vi "check out tracking state.vi"(6 "tick count":u32, 8 "ff vel?":bool, 9 "check out state":bool=TRUE, 10 "state number":u8, 11 "previous state":T1={"x state"={"pos estimate"=0.0, "v estimate"=0.0, "weighted position error sum"=0.0, "photon count"=0, "transmit tick count"=0, "axis number"=0, "px (levels^2)"=0.0, "pxv (levels^2/ticks)"=0.0, "pv (levels^2/ticks^2)"=0.0, "vel diff (levels^2/ticks^3)"=0.0, "gx"=0.0, "rtwiddle"=0.0, "photon count ch0"=0, "photon count ch1"=0, "Dx -levels^2/ticks"=0.0}, "y state"={"pos estimate"=0.0, "v estimate"=0.0, "weighted position error sum"=0.0, "photon count"=0, "transmit tick count"=0, "axis number"=1, "px (levels^2)"=0.0, "pxv (levels^2/ticks)"=0.0, "pv (levels^2/ticks^2)"=0.0, "vel diff (levels^2/ticks^3)"=0.0, "gx"=0.0, "rtwiddle"=0.0, "photon count ch0"=0, "photon count ch1"=0, "Dx -levels^2/ticks"=0.0}, "z state"={"pos estimate"=0.0, "v estimate"=0.0, "weighted position error sum"=0.0, "photon count"=0, "transmit tick count"=0, "axis number"=2, "px (levels^2)"=0.0, "pxv (levels^2/ticks)"=0.0, "pv (levels^2/ticks^2)"=0.0, "vel diff (levels^2/ticks^3)"=0.0, "gx"=0.0, "rtwiddle"=0.0, "photon count ch0"=0, "photon count ch1"=0, "Dx -levels^2/ticks"=0.0}, "spot number"=0}) -> (3 "state out":T1={"x state"={"pos estimate"=0.0, "v estimate"=0.0, "weighted position error sum"=0.0, "photon count"=0, "transmit tick count"=0, "axis number"=0, "px (levels^2)"=0.0, "pxv (levels^2/ticks)"=0.0, "pv (levels^2/ticks^2)"=0.0, "vel diff (levels^2/ticks^3)"=0.0, "gx"=0.0, "rtwiddle"=0.0, "photon count ch0"=0, "photon count ch1"=0, "Dx -levels^2/ticks"=0.0}, "y state"={"pos estimate"=0.0, "v estimate"=0.0, "weighted position error sum"=0.0, "photon count"=0, "transmit tick count"=0, "axis number"=1, "px (levels^2)"=0.0, "pxv (levels^2/ticks)"=0.0, "pv (levels^2/ticks^2)"=0.0, "vel diff (levels^2/ticks^3)"=0.0, "gx"=0.0, "rtwiddle"=0.0, "photon count ch0"=0, "photon count ch1"=0, "Dx -levels^2/ticks"=0.0}, "z state"={"pos estimate"=0.0, "v estimate"=0.0, "weighted position error sum"=0.0, "photon count"=0, "transmit tick count"=0, "axis number"=2, "px (levels^2)"=0.0, "pxv (levels^2/ticks)"=0.0, "pv (levels^2/ticks^2)"=0.0, "vel diff (levels^2/ticks^3)"=0.0, "gx"=0.0, "rtwiddle"=0.0, "photon count ch0"=0, "photon count ch1"=0, "Dx -levels^2/ticks"=0.0}, "spot number"=0})   [LabVIEW 2010]
uses:
  kalman 3-axis state.ctl
  integrating single axis kalman state.ctl
  <vilib>/rvi/DataTransferAndStorage/Container/XNode/niFpgaContainer.xnode
  <vilib>/rvi/Memory/Memory_Emulation/nirvimemoryEmulationManagerCache_GetValue.vi
  <vilib>/rvi/DataTransferAndStorage/Container/Common/niFpgaContainerGetUniqueNameForEmu.vi
  <vilib>/rvi/Memory/Memory_Emulation/nirvimemoryEmulationManagerCache_InsertValue.vi
  <vilib>/Utility/error.llb/Clear Errors.vi
  <vilib>/rvi/Memory/Memory_Emulation/nirvimemoryEmulationManagerCache_SetValue.vi
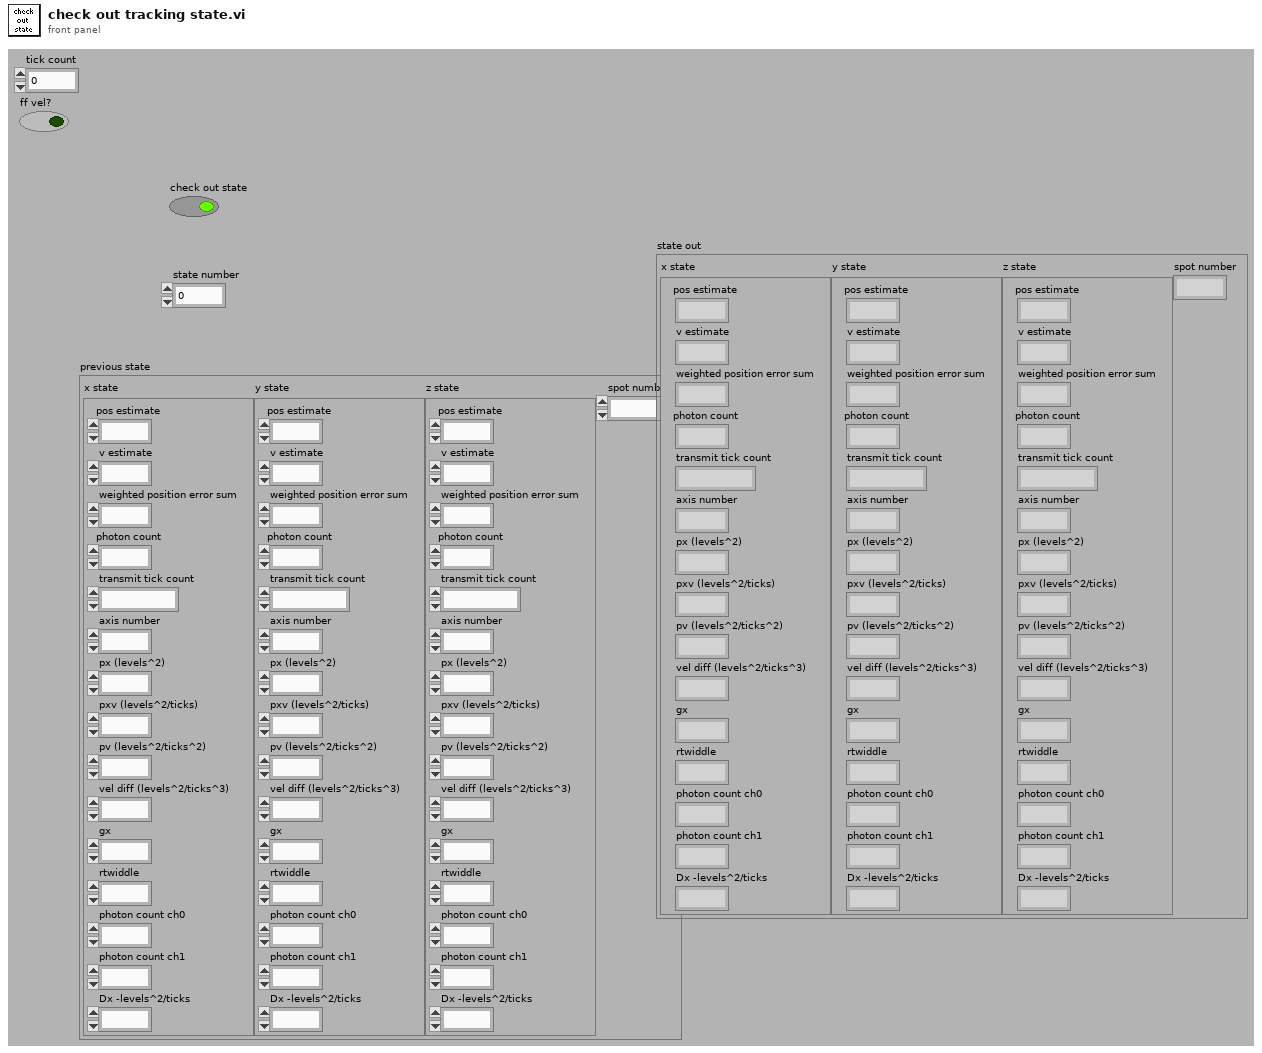
[diagram p1: front panel]
types:
  T1 = typedef "kalman 3-axis state.ctl" = cluster{"x state":T2, "y state":T2, "z state":T2, "spot number":u8}
  T2 = typedef "integrating single axis kalman state.ctl" = cluster{"pos estimate":fxp<+/-,32,16>, "v estimate":fxp<+/-,16,0>, "weighted position error sum":fxp<+/-,32,32>, "photon count":u32, "transmit tick count":u32, "axis number":u8, "px (levels^2)":fxp<+,32,19>, "pxv (levels^2/ticks)":fxp<+,32,2>, "pv (levels^2/ticks^2)":fxp<+,32,-14>, "vel diff (levels^2/ticks^3)":fxp<+,24,-22>, "gx":fxp<+,16,8>, "rtwiddle":fxp<+,16,26>, "photon count ch0":u32, "photon count ch1":u32, "Dx -levels^2/ticks":fxp<+,32,19>}
  T3 = cluster{"x state":cluster{"pos estimate":fxp<+/-,32,16>, "v estimate":fxp<+/-,16,0>, "weighted position error sum":fxp<+/-,32,32>, "photon count":u32, "transmit tick count":u32, "axis number":u8, "px (levels^2)":fxp<+,32,19>, "pxv (levels^2/ticks)":fxp<+,32,2>, "pv (levels^2/ticks^2)":fxp<+,32,-14>, "vel diff (levels^2/ticks^3)":fxp<+,24,-22>, "gx":fxp<+,16,8>, "rtwiddle":fxp<+,16,26>, "photon count ch0":u32, "photon count ch1":u32, "Dx - for pos only k-f":fxp<+,32,19>}, "y state":cluster{"pos estimate":fxp<+/-,32,16>, "v estimate":fxp<+/-,16,0>, "weighted position error sum":fxp<+/-,32,32>, "photon count":u32, "transmit tick count":u32, "axis number":u8, "px (levels^2)":fxp<+,32,19>, "pxv (levels^2/ticks)":fxp<+,32,2>, "pv (levels^2/ticks^2)":fxp<+,32,-14>, "vel diff (levels^2/ticks^3)":fxp<+,24,-22>, "gx":fxp<+,16,8>, "rtwiddle":fxp<+,16,26>, "photon count ch0":u32, "photon count ch1":u32, "Dx - for pos only k-f":fxp<+,32,19>}, "z state":cluster{"pos estimate":fxp<+/-,32,16>, "v estimate":fxp<+/-,16,0>, "weighted position error sum":fxp<+/-,32,32>, "photon count":u32, "transmit tick count":u32, "axis number":u8, "px (levels^2)":fxp<+,32,19>, "pxv (levels^2/ticks)":fxp<+,32,2>, "pv (levels^2/ticks^2)":fxp<+,32,-14>, "vel diff (levels^2/ticks^3)":fxp<+,24,-22>, "gx":fxp<+,16,8>, "rtwiddle":fxp<+,16,26>, "photon count ch0":u32, "photon count ch1":u32, "Dx - for pos only k-f":fxp<+,32,19>}, "spot number":u8}
  T4 = cluster{"pos estimate":fxp<+/-,32,16>, "v estimate":fxp<+/-,16,0>, "weighted position error sum":fxp<+/-,32,32>, "photon count":u32, "transmit tick count":u32, "axis number":u8, "px (levels^2)":fxp<+,32,19>, "pxv (levels^2/ticks)":fxp<+,32,2>, "pv (levels^2/ticks^2)":fxp<+,32,-14>, "vel diff (levels^2/ticks^3)":fxp<+,24,-22>, "gx":fxp<+,16,8>, "rtwiddle":fxp<+,16,26>, "photon count ch0":u32, "photon count ch1":u32, "Dx - for pos only k-f":fxp<+,32,19>}
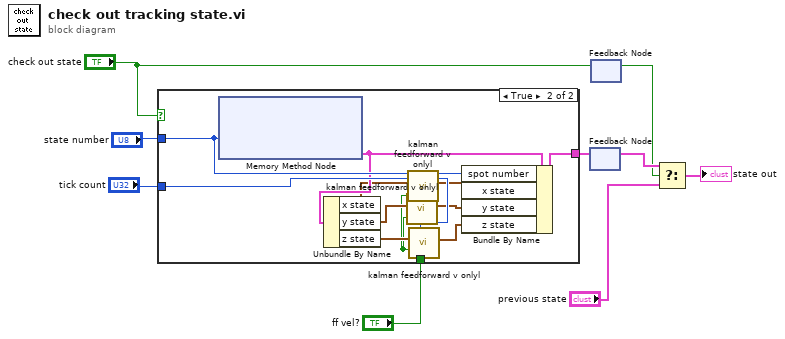
[diagram p0: block diagram]
diagram:
  n1 = case shown="True" "check out state" {
    tunnel: "state number" -> [_ w20]
    tunnel: "tick count" -> [_ w19]
    tunnel: [_ w18] -> w7
    tunnel: "ff vel?" -> [_ w10]
    frame False {
    }
    frame True {
      n2 = xnode ("Memory Method Node")("Address"=w20) -> ("Data"=w17:T3)  [unwired: 1 in, 1 out]
      n3 = Unbundle By Name(w17) -> ("x state"=w16:T4, "y state"=w15:T4, "z state"=w14:T4)
      n4 = call "kalman feedforward v onlyl.vi"("ff vel?"=w10, "tick count"=w19, "state in"=w15) -> ("state out"=w12:T2)  [unwired: 8 in]
      n5 = call "kalman feedforward v onlyl.vi"("ff vel?"=w10, "tick count"=w19, "state in"=w16) -> ("state out"=w13:T2)  [unwired: 8 in]
      n6 = call "kalman feedforward v onlyl.vi"("ff vel?"=w10, "tick count"=w19, "state in"=w14) -> ("state out"=w11:T2)  [unwired: 8 in]
      n7 = Bundle By Name(cluster=w17, "spot number"=w20, "x state"=w13, "y state"=w12, "z state"=w11) -> (w18:T3)
    }
  }
  n8 = feedback-in #1(w7) -> ()
  n9 = feedback #1() -> (w6:T3)  [unwired: 1 in]
  n10 = feedback #2() -> (w2:bool)  [unwired: 1 in]
  n11 = feedback-in #2("check out state") -> ()
  n12 = Select(t=w6, s=w2, f="previous state") -> (s? t:f=→"state out":T1)
